vi "testingauto.vi"() -> ()   [LabVIEW 2014]
uses:
  <vilib>/vision/NI_Vision_Development_Module.lvlib
  <instrlib>/KD Scientific 2XX Series/KD Scientific 2XX Series.lvlib
panel:
  in  "Number of Cycles":i32
  in  "Min Pressure":dbl
  in  "Max Pressure":dbl
  out "Status":T1
  in  "stop 2":bool
  out "Delivered Volume":dbl
  out "Units":string
  in  "Baud Rate (9600)":u32(ring)=9600 items=["300"=300, "1200"=1200, "2400"=2400, "4800"=4800, "9600"=9600]
  in  "Withdrawal Settings":T2={"Flow Rate (5)"=5.0, "Volume (10)"=10.0, "Volume Units (ml)"=enum."milliliters (ml)", "Rate Units (ml/min.)"=enum."milliliters per minute (ml/min.)"} {"Volume (10)" format="%#.3g"}
  in  "Diameter (8.75 mm)":dbl=8.75
  in  "Infusion Settings":T2={"Flow Rate (5)"=5.0, "Volume (10)"=10.0, "Volume Units (ml)"=enum."milliliters (ml)", "Rate Units (ml/min.)"=enum."milliliters per minute (ml/min.)"}
  in  "Address (0)":i32 format="%0.0f"
  in  "error in (no error)":errorcluster
  in  "VISA resource name":refnum<visa-resource-name>="COM1"
  in  "stop":bool
  out "Image":T3(plugin-control)
  out "Particle Measurements (Pixels) (Particle Analysis 1)":dbl[][](array[numeric]) format="%.2f"
  out "subarray":dbl[](array[numeric])
  out "The diameter":dbl[](array[numeric])
  in  "stop (F)":bool
  out "Data from Transducer":dynamicdata(graph) caption="Voltage from Transducer V"
  out "Voltage from pressure transducer":dbl[](array[numeric])
  out "Pressure mm Hg":dbl[](graph)
  in  "Calibration factor":dbl[](array[numeric])
  in  "Zero Error":dbl[](array[numeric])
  out "pressure mm Hg":dbl[](array[numeric])
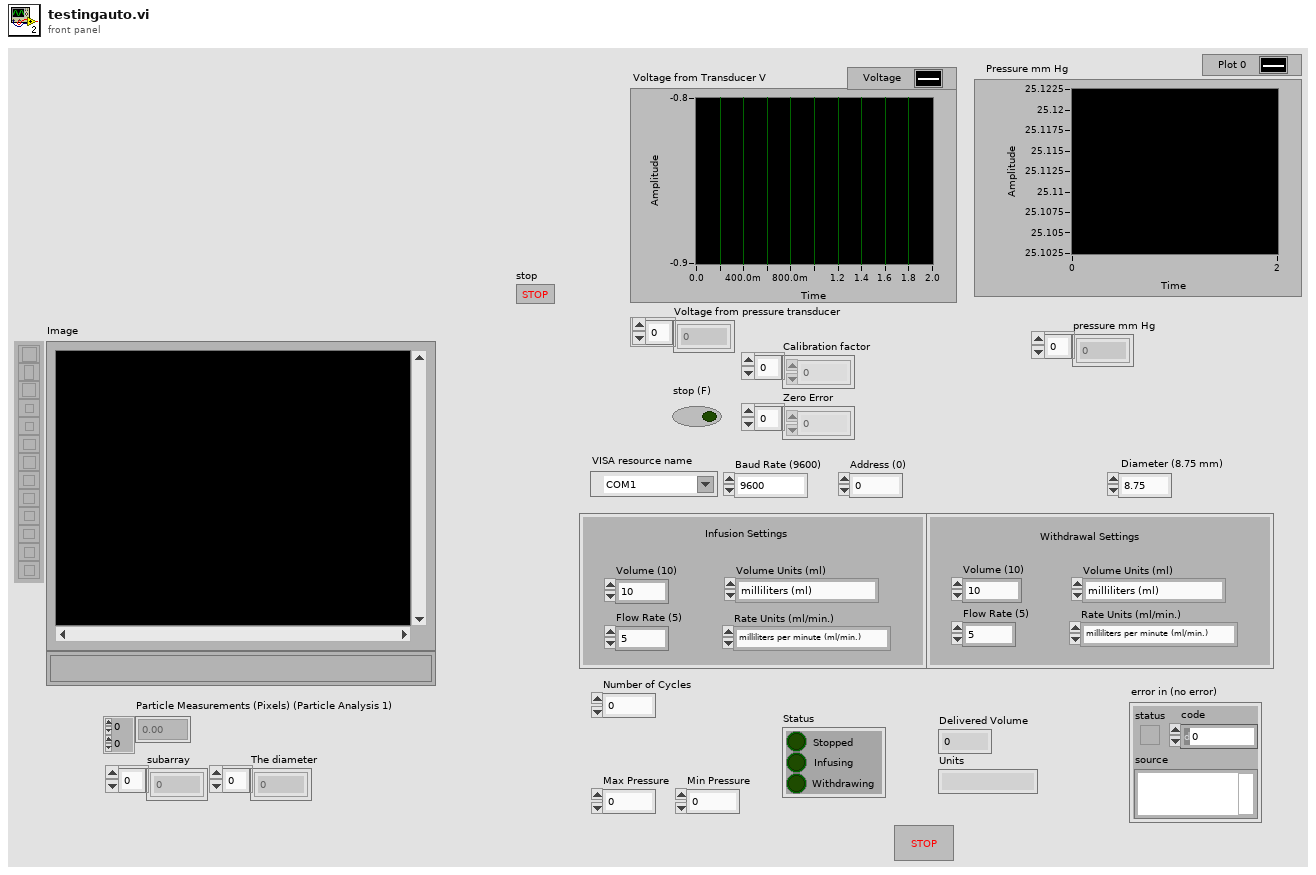
[diagram p1: front panel]
types:
  T1 = cluster{"Stopped":bool, "Infusing":bool, "Withdrawing":bool}
  T2 = cluster{"Flow Rate (5)":dbl, "Volume (10)":dbl, "Volume Units (ml)":enum16{"milliliters (ml)", "microliters (ul)"}, "Rate Units (ml/min.)":enum16{"milliliters per minute (ml/min.)", "milliliters per hour (ml/hr.)", "microliters per minute (ul/min.)", "microliters per hour (ul/hr.)"}}
  T3 = typedef "IMAQ Image.ctl" = refnum<image>
  T4 = typedef "Board Id" = u8
  T5 = typedef "ROI Descriptor" = cluster{"Global Rectangle":i32[], "Contours":cluster{"ID":enum32{"External", "Internal"}, "Type":u32, "Coordinates":i32[]}[]}
  T6 = enum16{"milliliters per minute (ml/min.)", "milliliters per hour (ml/hr.)", "microliters per minute (ul/min.)", "microliters per hour (ul/hr.)"}
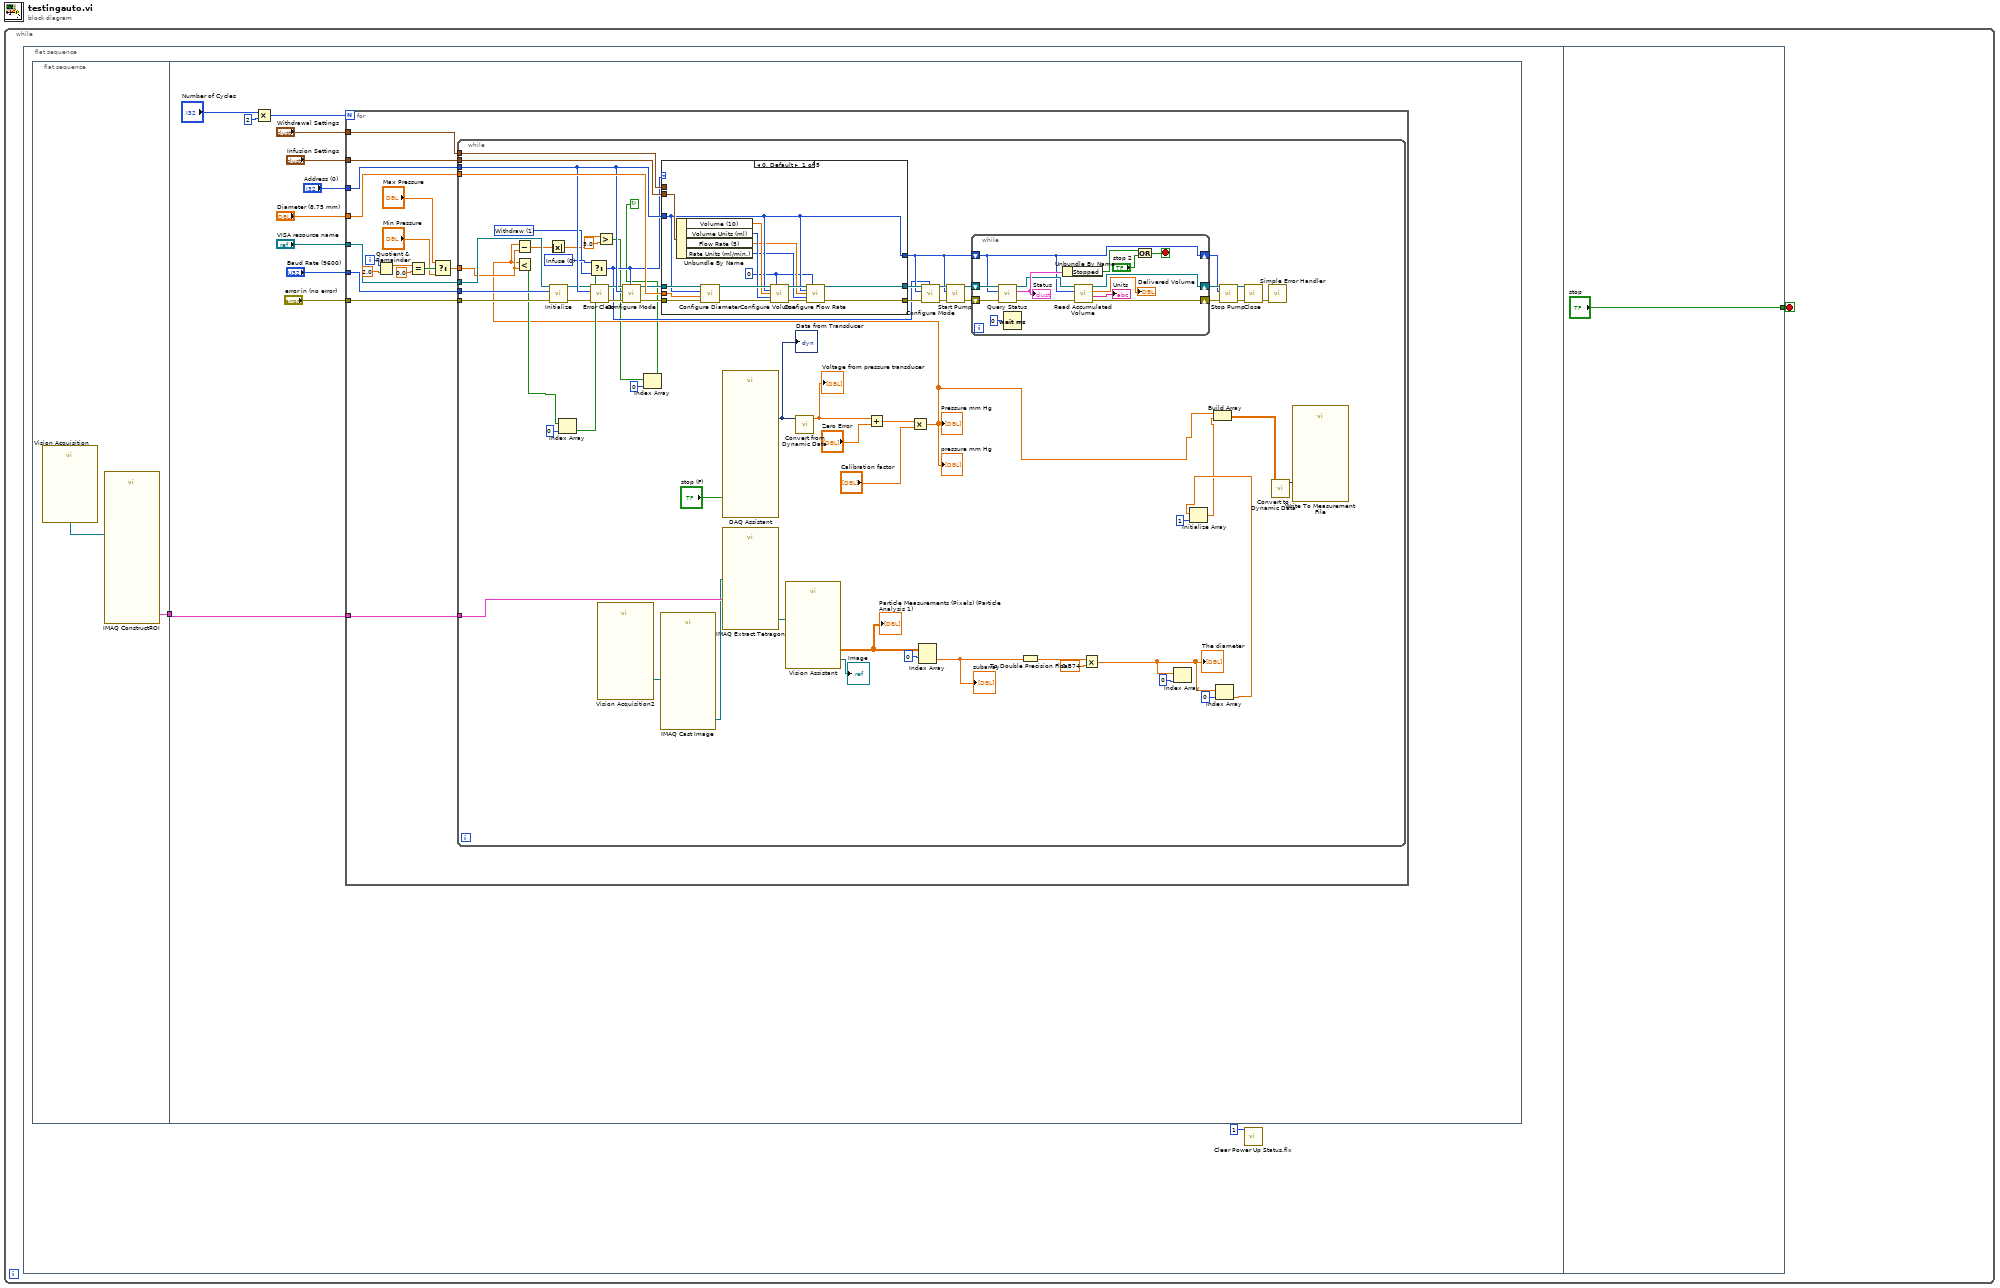
[diagram p0: block diagram]
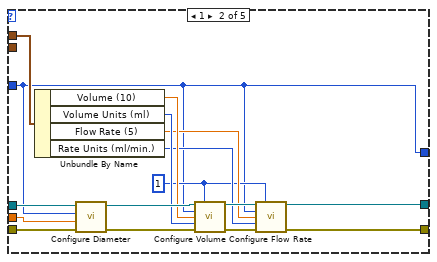
[diagram p2: hidden frame]
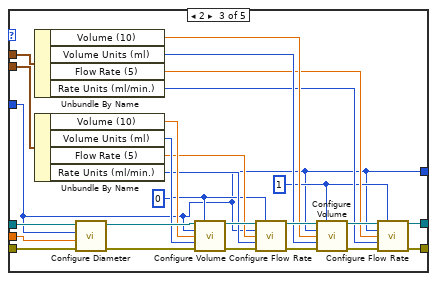
[diagram p3: hidden frame]
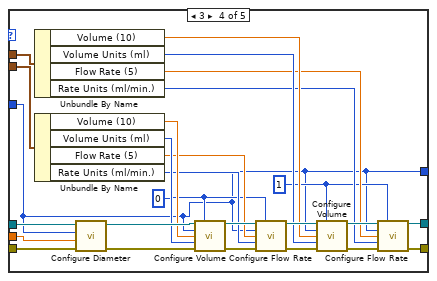
[diagram p4: hidden frame]
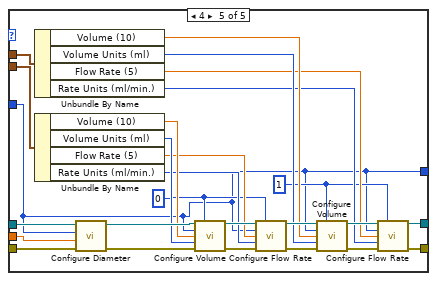
[diagram p5: hidden frame]
diagram:
  n1 = while {
    stop <- w1 stop-if-true
    n2 = flat-sequence {
      tunnel: ["stop"] -> w1
      frame #0 {
        n3 = flat-sequence {
          tunnel: [w4] -> w3
          tunnel: w3 -> [w6]
          frame #0 {
            n4 = call "Vision Acquisition"() -> ("Image Out"=w5:T3)  [unwired: 26 in, 1 out]
            n5 = call "IMAQ ConstructROI"("Image"=w5) -> ("ROI Descriptor Out"=w4:T5)  [unwired: 7 in, 3 out]
          }
          frame #1 {
            n6 = Multiply(x="Number of Cycles", y=2) -> (x*y=w16:i32)
            n7 = for {
              N: w16 -> [_]
              tunnel: "VISA resource name" -> [w32]
              tunnel: "error in (no error)" -> [w31]
              tunnel: "Infusion Settings" -> [w30]
              tunnel: "Withdrawal Settings" -> [w29]
              tunnel: "Diameter (8.75 mm)" -> [w28]
              tunnel: "Baud Rate (9600)" -> [w27]
              tunnel: "Address (0)" -> [w26]
              tunnel: w6 -> [w17]
              i -> [w24]
              n8 = Quotient & Remainder(x=w24, y=2.0) -> (x-y*floor(x/y)=w22:dbl)  [unwired: 1 out]
              n9 = Equal?(x=w22, y=0.0) -> (x = y?=w21:bool)
              n10 = Select(t="Max Pressure", s=w21, f="Min Pressure") -> (s? t:f=w18:dbl)
              n11 = while {
                tunnel: w32 -> [w96]
                tunnel: w31 -> [w95]
                tunnel: w30 -> [w94]
                tunnel: w29 -> [w93]
                tunnel: w28 -> [w92]
                tunnel: w27 -> [w91]
                tunnel: w26 -> [w90]
                tunnel: w18 -> [w67]
                tunnel: w17 -> [w40]
                stop <- w52 continue-if-true
                w69 = u16 1 items=["Withdraw"=1]
                w70 = u16 0 items=["Infuse"] ("Mode (infuse)")
                n12 = call <instrlib>:"Initialize.vi"("error in (no error)"=w95, "Baud Rate (9600)"=w91, "VISA resource name"=w96) -> ("error out"=w72:errorcluster, "VISA resource name out"=w71:refnum<visa-resource-name>)  [unwired: 7 in]
                n13 = call <instrlib>:"Error Clear.vi"("error in (no error)"=w72, "Address (0)"=w90, "VISA resource name"=w71) -> ("error out"=w73:errorcluster, "VISA resource name out"=w74:refnum<visa-resource-name>)  [unwired: 6 in, 1 out]
                n14 = call "Vision Acquisition2"() -> ("Image Out"=w49:T3)  [unwired: 25 in, 2 out]
                n15 = call "IMAQ Cast Image"("Image Src"=w49) -> ("Image Dst Out"=w39:T3)  [unwired: 9 in, 1 out]
                n16 = call "DAQ Assistant"("stop (F)"="stop (F)") -> ("data"=w58:dynamicdata)  [unwired: 15 in, 3 out]
                "Data from Transducer" <- w58
                n17 = call-poly "IMAQ Extract Tetragon"("ROI Descriptor"=w40, "Image Src"=w39) -> ("Image Dst Out"=w42:T3)  [unwired: 8 in, 1 out]
                n18 = call "Vision Assistant"("Image In"=w42) -> ("Image Out"=→"Image":T3, "Particle Measurements (Pixels) (Particle Analysis 1)"=w43:dbl[][])  [unwired: 23 in, 2 out]
                "Particle Measurements (Pixels) (Particle Analysis 1)" <- w43
                n19 = call "Convert from Dynamic Data"("Dynamic Data Type"=w58) -> ("Array"=w61:dbl[])  [unwired: 3 in]
                "Voltage from pressure transducer" <- w61
                n20 = Add(x=w61, y="Zero Error") -> (x+y=w59:dbl[])
                n21 = Multiply(x=w59, y="Calibration factor") -> (x*y=w37:dbl[])
                "Pressure mm Hg" <- w37
                "pressure mm Hg" <- w37
                n22 = Subtract(x=w37, y=w67) -> (x-y=w66:dbl[])
                n23 = Less?(x=w37, y=w67) -> (x < y?=w57:bool[])
                n24 = Absolute Value(x=w66) -> (abs(x)=w65:dbl[])
                n25 = Index Array(array=w57, index=0) -> (element=w55:bool)
                n26 = Select(t=w70, s=w55, f=w69) -> (s? t:f=w68:u16)
                n27 = Greater?(x=w65, y=5.0) -> (0:w54:bool[])
                n28 = call <instrlib>:"Configure Mode.vi"("Mode (infuse)"=w68, "error in (no error)"=w73, "Address (0)"=w90, "VISA resource name"=w74) -> ("error out"=w76:errorcluster, "VISA resource name out"=w75:refnum<visa-resource-name>)  [unwired: 6 in]
                n29 = Index Array(array=w54, index=0) -> (element=w52:bool)
                n30 = case shown="0, Default" w68 {
                  tunnel: w94 -> [w106 _ w154 w180 w206]
                  tunnel: w93 -> [_ w128 w153 w179 w205]
                  tunnel: w75 -> [w112 w127 w152 w178 w204]
                  tunnel: w76 -> [w111 w123 w151 w177 w203]
                  tunnel: w92 -> [w105 w119 w134 w160 w186]
                  tunnel: [w104 w113 w129 w155 w181] -> w77
                  tunnel: w90 -> [w104 w113 w129 w155 w181]
                  tunnel: [w99 w124 w131 w157 w183] -> w81
                  tunnel: [w98 w120 w130 w156 w182] -> w80
                  frame 0, Default {
                    w97 = 0
                    n31 = Unbundle By Name(w106) -> ("Volume (10)"=w103:dbl, "Volume Units (ml)"=w102:enum16{"milliliters (ml)", "microliters (ul)"}, "Flow Rate (5)"=w101:dbl, "Rate Units (ml/min.)"=w100:T6)
                    n32 = call <instrlib>:"Configure Diameter.vi"("error in (no error)"=w111, "Diameter (8.75 mm)"=w105, "Address (0)"=w104, "VISA resource name"=w112) -> ("error out"=w109:errorcluster, "VISA resource name out"=w110:refnum<visa-resource-name>)  [unwired: 6 in]
                    n33 = call <instrlib>:"Configure Volume.vi"("VISA resource name"=w110, "Mode (infuse)"=w97, "Address (0)"=w104, "Volume (100)"=w103, "Units (0: milliliters)"=w102, "error in (no error)"=w109) -> ("VISA resource name out"=w108:refnum<visa-resource-name>, "error out"=w107:errorcluster)  [unwired: 8 in]
                    n34 = call <instrlib>:"Configure Flow Rate.vi"("VISA resource name"=w108, "Mode (infuse)"=w97, "Address (0)"=w104, "Flow Rate (5)"=w101, "Units (0: milliliters per minute)"=w100, "error in (no error)"=w107) -> ("VISA resource name out"=w99:refnum<visa-resource-name>, "error out"=w98:errorcluster)  [unwired: 8 in]
                  }
                  frame 1 {
                    w114 = 1
                    n35 = Unbundle By Name(w128) -> ("Volume (10)"=w118:dbl, "Volume Units (ml)"=w117:enum16{"milliliters (ml)", "microliters (ul)"}, "Flow Rate (5)"=w116:dbl, "Rate Units (ml/min.)"=w115:T6)
                    n36 = call <instrlib>:"Configure Diameter.vi"("error in (no error)"=w123, "Diameter (8.75 mm)"=w119, "Address (0)"=w113, "VISA resource name"=w127) -> ("error out"=w122:errorcluster, "VISA resource name out"=w126:refnum<visa-resource-name>)  [unwired: 6 in]
                    n37 = call <instrlib>:"Configure Volume.vi"("VISA resource name"=w126, "Mode (infuse)"=w114, "Address (0)"=w113, "Volume (100)"=w118, "Units (0: milliliters)"=w117, "error in (no error)"=w122) -> ("VISA resource name out"=w125:refnum<visa-resource-name>, "error out"=w121:errorcluster)  [unwired: 8 in]
                    n38 = call <instrlib>:"Configure Flow Rate.vi"("VISA resource name"=w125, "Mode (infuse)"=w114, "Address (0)"=w113, "Flow Rate (5)"=w116, "Units (0: milliliters per minute)"=w115, "error in (no error)"=w121) -> ("VISA resource name out"=w124:refnum<visa-resource-name>, "error out"=w120:errorcluster)  [unwired: 8 in]
                  }
                  frame 2 {
                    w132 = 1
                    w133 = 0
                    n39 = Unbundle By Name(w153) -> ("Volume (10)"=w138:dbl, "Volume Units (ml)"=w137:enum16{"milliliters (ml)", "microliters (ul)"}, "Flow Rate (5)"=w136:dbl, "Rate Units (ml/min.)"=w135:T6)
                    n40 = Unbundle By Name(w154) -> ("Volume (10)"=w142:dbl, "Volume Units (ml)"=w141:enum16{"milliliters (ml)", "microliters (ul)"}, "Flow Rate (5)"=w140:dbl, "Rate Units (ml/min.)"=w139:T6)
                    n41 = call <instrlib>:"Configure Diameter.vi"("error in (no error)"=w151, "Diameter (8.75 mm)"=w134, "Address (0)"=w129, "VISA resource name"=w152) -> ("error out"=w146:errorcluster, "VISA resource name out"=w150:refnum<visa-resource-name>)  [unwired: 6 in]
                    n42 = call <instrlib>:"Configure Volume.vi"("VISA resource name"=w150, "Mode (infuse)"=w133, "Address (0)"=w129, "Volume (100)"=w142, "Units (0: milliliters)"=w141, "error in (no error)"=w146) -> ("VISA resource name out"=w149:refnum<visa-resource-name>, "error out"=w145:errorcluster)  [unwired: 8 in]
                    n43 = call <instrlib>:"Configure Flow Rate.vi"("VISA resource name"=w149, "Mode (infuse)"=w133, "Address (0)"=w129, "Flow Rate (5)"=w140, "Units (0: milliliters per minute)"=w139, "error in (no error)"=w145) -> ("VISA resource name out"=w148:refnum<visa-resource-name>, "error out"=w144:errorcluster)  [unwired: 8 in]
                    n44 = call <instrlib>:"Configure Volume.vi"("VISA resource name"=w148, "Mode (infuse)"=w132, "Address (0)"=w129, "Volume (100)"=w138, "Units (0: milliliters)"=w137, "error in (no error)"=w144) -> ("VISA resource name out"=w147:refnum<visa-resource-name>, "error out"=w143:errorcluster)  [unwired: 8 in]
                    n45 = call <instrlib>:"Configure Flow Rate.vi"("VISA resource name"=w147, "Mode (infuse)"=w132, "Address (0)"=w129, "Flow Rate (5)"=w136, "Units (0: milliliters per minute)"=w135, "error in (no error)"=w143) -> ("VISA resource name out"=w131:refnum<visa-resource-name>, "error out"=w130:errorcluster)  [unwired: 8 in]
                  }
                  frame 3 {
                    w158 = 1
                    w159 = 0
                    n46 = Unbundle By Name(w179) -> ("Volume (10)"=w164:dbl, "Volume Units (ml)"=w163:enum16{"milliliters (ml)", "microliters (ul)"}, "Flow Rate (5)"=w162:dbl, "Rate Units (ml/min.)"=w161:T6)
                    n47 = Unbundle By Name(w180) -> ("Volume (10)"=w168:dbl, "Volume Units (ml)"=w167:enum16{"milliliters (ml)", "microliters (ul)"}, "Flow Rate (5)"=w166:dbl, "Rate Units (ml/min.)"=w165:T6)
                    n48 = call <instrlib>:"Configure Diameter.vi"("error in (no error)"=w177, "Diameter (8.75 mm)"=w160, "Address (0)"=w155, "VISA resource name"=w178) -> ("error out"=w172:errorcluster, "VISA resource name out"=w176:refnum<visa-resource-name>)  [unwired: 6 in]
                    n49 = call <instrlib>:"Configure Volume.vi"("VISA resource name"=w176, "Mode (infuse)"=w159, "Address (0)"=w155, "Volume (100)"=w168, "Units (0: milliliters)"=w167, "error in (no error)"=w172) -> ("VISA resource name out"=w175:refnum<visa-resource-name>, "error out"=w171:errorcluster)  [unwired: 8 in]
                    n50 = call <instrlib>:"Configure Flow Rate.vi"("VISA resource name"=w175, "Mode (infuse)"=w159, "Address (0)"=w155, "Flow Rate (5)"=w166, "Units (0: milliliters per minute)"=w165, "error in (no error)"=w171) -> ("VISA resource name out"=w174:refnum<visa-resource-name>, "error out"=w170:errorcluster)  [unwired: 8 in]
                    n51 = call <instrlib>:"Configure Volume.vi"("VISA resource name"=w174, "Mode (infuse)"=w158, "Address (0)"=w155, "Volume (100)"=w164, "Units (0: milliliters)"=w163, "error in (no error)"=w170) -> ("VISA resource name out"=w173:refnum<visa-resource-name>, "error out"=w169:errorcluster)  [unwired: 8 in]
                    n52 = call <instrlib>:"Configure Flow Rate.vi"("VISA resource name"=w173, "Mode (infuse)"=w158, "Address (0)"=w155, "Flow Rate (5)"=w162, "Units (0: milliliters per minute)"=w161, "error in (no error)"=w169) -> ("VISA resource name out"=w157:refnum<visa-resource-name>, "error out"=w156:errorcluster)  [unwired: 8 in]
                  }
                  frame 4 {
                    w184 = 1
                    w185 = 0
                    n53 = Unbundle By Name(w205) -> ("Volume (10)"=w190:dbl, "Volume Units (ml)"=w189:enum16{"milliliters (ml)", "microliters (ul)"}, "Flow Rate (5)"=w188:dbl, "Rate Units (ml/min.)"=w187:T6)
                    n54 = Unbundle By Name(w206) -> ("Volume (10)"=w194:dbl, "Volume Units (ml)"=w193:enum16{"milliliters (ml)", "microliters (ul)"}, "Flow Rate (5)"=w192:dbl, "Rate Units (ml/min.)"=w191:T6)
                    n55 = call <instrlib>:"Configure Diameter.vi"("error in (no error)"=w203, "Diameter (8.75 mm)"=w186, "Address (0)"=w181, "VISA resource name"=w204) -> ("error out"=w198:errorcluster, "VISA resource name out"=w202:refnum<visa-resource-name>)  [unwired: 6 in]
                    n56 = call <instrlib>:"Configure Volume.vi"("VISA resource name"=w202, "Mode (infuse)"=w185, "Address (0)"=w181, "Volume (100)"=w194, "Units (0: milliliters)"=w193, "error in (no error)"=w198) -> ("VISA resource name out"=w201:refnum<visa-resource-name>, "error out"=w197:errorcluster)  [unwired: 8 in]
                    n57 = call <instrlib>:"Configure Flow Rate.vi"("VISA resource name"=w201, "Mode (infuse)"=w185, "Address (0)"=w181, "Flow Rate (5)"=w192, "Units (0: milliliters per minute)"=w191, "error in (no error)"=w197) -> ("VISA resource name out"=w200:refnum<visa-resource-name>, "error out"=w196:errorcluster)  [unwired: 8 in]
                    n58 = call <instrlib>:"Configure Volume.vi"("VISA resource name"=w200, "Mode (infuse)"=w184, "Address (0)"=w181, "Volume (100)"=w190, "Units (0: milliliters)"=w189, "error in (no error)"=w196) -> ("VISA resource name out"=w199:refnum<visa-resource-name>, "error out"=w195:errorcluster)  [unwired: 8 in]
                    n59 = call <instrlib>:"Configure Flow Rate.vi"("VISA resource name"=w199, "Mode (infuse)"=w184, "Address (0)"=w181, "Flow Rate (5)"=w188, "Units (0: milliliters per minute)"=w187, "error in (no error)"=w195) -> ("VISA resource name out"=w183:refnum<visa-resource-name>, "error out"=w182:errorcluster)  [unwired: 8 in]
                  }
                }
                n60 = Index Array(array=w43, index (row)=0) -> (element=w45:dbl[])  [unwired: 1 in]
                "subarray" <- w45
                n61 = call <instrlib>:"Configure Mode.vi"("Mode (infuse)"=w68, "error in (no error)"=w80, "Address (0)"=w77, "VISA resource name"=w81) -> ("error out"=w78:errorcluster, "VISA resource name out"=w79:refnum<visa-resource-name>)  [unwired: 6 in]
                n62 = call <instrlib>:"Start Pump.vi"("error in (no error)"=w78, "Address (0)"=w77, "VISA resource name"=w79) -> ("error out"=w88:errorcluster, "VISA resource name out"=w89:refnum<visa-resource-name>)  [unwired: 7 in]
                n63 = while {
                  shift-right: [w209] -> w85
                  shift-left: w77 -> [w209]
                  shift-right: [w211] -> w87
                  shift-left: w89 -> [w217]
                  shift-right: [w210] -> w86
                  shift-left: w88 -> [w218]
                  stop <- w215 stop-if-true
                  n64 = call <instrlib>:"Query Status.vi"("error in (no error)"=w218, "Address (0)"=w209, "VISA resource name"=w217) -> ("error out"=w220:errorcluster, "Status"=w216:T1, "VISA resource name out"=w212:refnum<visa-resource-name>)  [unwired: 6 in]
                  "Status" <- w216
                  n65 = Wait (ms)(milliseconds to wait=u32 0) -> ()  [unwired: 1 out]
                  n66 = Unbundle By Name(w216) -> ("Stopped"=w214:bool)
                  n67 = call <instrlib>:"Read Accumulated Volume.vi"("error in (no error)"=w220, "Address (0)"=w209, "VISA resource name"=w212) -> ("error out"=w210:errorcluster, "Units"=→"Units":string, "Delivered Volume"=→"Delivered Volume":dbl, "VISA resource name out"=w211:refnum<visa-resource-name>)  [unwired: 5 in]
                  n68 = Or(x=w214, y="stop 2") -> (x .or. y?=w215:bool)
                }
                n69 = To Double Precision Float(number=w45) -> (double precision float=w46:dbl[])
                n70 = Multiply(x=w46, y=0.374) -> (x*y=w51:dbl[])
                "The diameter" <- w51
                n71 = Index Array(array=w51, index=0) -> ()  [unwired: 1 out]
                n72 = Index Array(array=w51, index=0) -> (element=w36:dbl)
                n73 = Initialize Array(w36, 1 ("dimension size")) -> (w35:dbl[])
                n74 = Build Array(w37, w35) -> (w34:dbl[][])
                n75 = call <instrlib>:"Stop Pump.vi"("error in (no error)"=w86, "Address (0)"=w85, "VISA resource name"=w87) -> ("error out"=w83:errorcluster, "VISA resource name out"=w82:refnum<visa-resource-name>)  [unwired: 7 in]
                n76 = call <instrlib>:"Close.vi"("error in (no error)"=w83, "VISA resource name"=w82) -> ("error out"=w84:errorcluster)  [unwired: 9 in]
                n77 = call <vilib>:"Simple Error Handler.vi"("error in (no error)"=w84) -> ()  [unwired: 4 in, 5 out]
                n78 = call "Convert to Dynamic Data"("2D Array"=w34) -> ("Dynamic Data Type"=w33:dynamicdata)  [unwired: 3 in]
                n79 = call "Write To Measurement File"("Signals"=w33) -> ()  [unwired: 16 in, 3 out]
              }
            }
          }
        }
        n80 = call <vilib>:"Clear Power Up Status.flx"("Board ID"=T4 1) -> ()  [unwired: 6 in, 2 out]
      }
      frame #1 {
      }
    }
  }
